vi "MarbleController.vi"   [LabVIEW 2016]
uses:
  <vilib>/NXT/Block Support/NXT_InputPort.ctl
  <vilib>/NXT/Block Support/NXT_OutputPort.ctl
  <vilib>/NXT/Dual Mode Library/Sensors/Touch_Count.vi
  <vilib>/NXT/NXTIO Xnodes/NXTIONodeSubVIs/NXTMoveMotors.vi
  <vilib>/NXT/NXTIO Xnodes/NXTIONodeSubVIs/NXTStopMotors.vi
  <vilib>/NXT/NXTIO Xnodes/NXTIONodeSubVIs/NXTMotorRunDistance.vi
  <vilib>/NXT/NXTIO Xnodes/AddressXNode/NXTIOAddress.xnode
  <vilib>/NXT/NXTIO Xnodes/NXTIOXNode/NXTIO.xnode
  <vilib>/NXT/Subs/LVHSConnector.ctl
  <vilib>/NXT/LegoClasses/BrickReference/BrickReference.lvclass
types:
  T1 = typedef "NXT_OutputPort.ctl" = u8
  T2 = typedef "NXT_InputPort.ctl" = u32
  T3 = typedef "LVHSConnector.ctl" = refnum<class "BrickReference.lvclass">
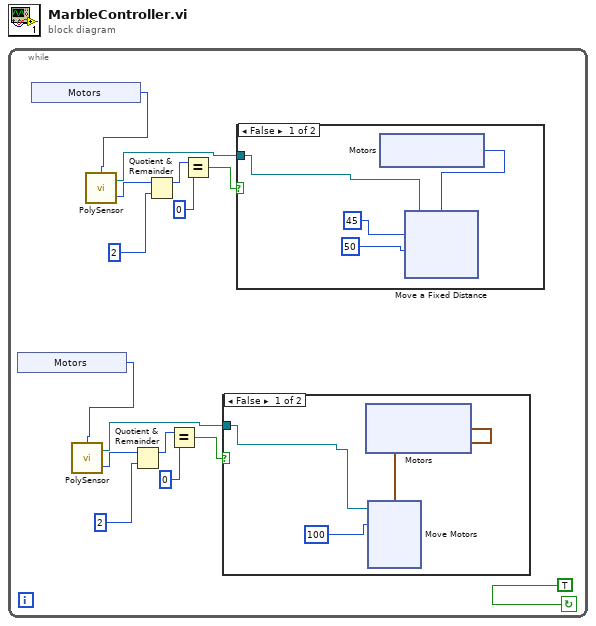
[diagram p0: block diagram]
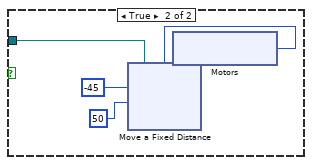
[diagram p2: hidden frame]
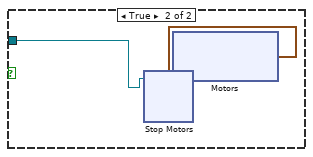
[diagram p3: hidden frame]
diagram:
  n1 = while {
    stop <- TRUE continue-if-true
    n2 = xnode "Motors"() -> ("Sensor"=w8:T2)
    n3 = xnode "Motors"() -> ("Sensor"=w1:T2)
    n4 = call-poly <vilib>:"PolySensor.vi"("Port (Port 1)"=w8) -> ("Count"=w14:i16, "NXT/EV3"=w9:T3)  [unwired: 2 in]
    n5 = call-poly <vilib>:"PolySensor.vi"("Port (Port 1)"=w1) -> ("Count"=w7:i16, "NXT/EV3"=w2:T3)  [unwired: 2 in]
    n6 = Quotient & Remainder(x=w14, y=2) -> (x-y*floor(x/y)=w12:i32)  [unwired: 1 out]
    n7 = Quotient & Remainder(x=w7, y=2) -> (x-y*floor(x/y)=w5:i32)  [unwired: 1 out]
    n8 = Equal?(x=w12, y=0) -> (x = y?=w10:bool)
    n9 = Equal?(x=w5, y=0) -> (x = y?=w3:bool)
    n10 = case shown="False" w10 {
      tunnel: w9 -> [w50 w61]
      frame False {
        n11 = xnode "Motors"() -> ("Motor"=w49:cluster{"Port":T1, "Port":T1})
        n12 = xnode "Move Motors"("Power/Speed 1"=100, "Motors"=w49, "NXT/EV3"=w50) -> ()  [unwired: 1 in, 1 out]
      }
      frame True {
        n13 = xnode "Motors"() -> ("Motor"=w60:cluster{"Port":T1, "Port":T1})
        n14 = xnode "Stop Motors"("Motors"=w60, "NXT/EV3"=w61) -> ()  [unwired: 1 out]
      }
    }
    n15 = case shown="False" w3 {
      tunnel: w2 -> [w19 w35]
      frame False {
        n16 = xnode "Motors"() -> ("Motor"=w20:T1)
        n17 = xnode "Move a Fixed Distance"("Speed 1"=50, "Distance 1"=45, "Motors"=w20, "NXT/EV3"=w19) -> ()  [unwired: 1 out]
      }
      frame True {
        n18 = xnode "Motors"() -> ("Motor"=w34:T1)
        n19 = xnode "Move a Fixed Distance"("Speed 1"=50, "Distance 1"=-45, "Motors"=w34, "NXT/EV3"=w35) -> ()  [unwired: 1 out]
      }
    }
  }
